vi "Load Matrix.vi"(7 "section":string, 8 "error in (no error) 2":errorcluster, 10 "refnum in":T2, 11 "Keys":string[](array[string])) -> (0 "error in (no error)":errorcluster, 1 "Matrix 2":dbl[][](array[numeric]), 2 "Matrix 1":dbl[][](array[numeric]), 3 "refnum out":T2)   [LabVIEW 2013]
uses:
  <vilib>/Utility/config.llb/Config Data RefNum.ctl
  Metadata/LBCB Number.ctl
  <vilib>/Utility/config.llb/Read Key (String).vi
  <vilib>/Utility/config.llb/NI_LVConfig.lvlib
panel:
  out "key names":string[](array[string])
  in  "LBCB Number":T1
  in  "delimiter":string="."
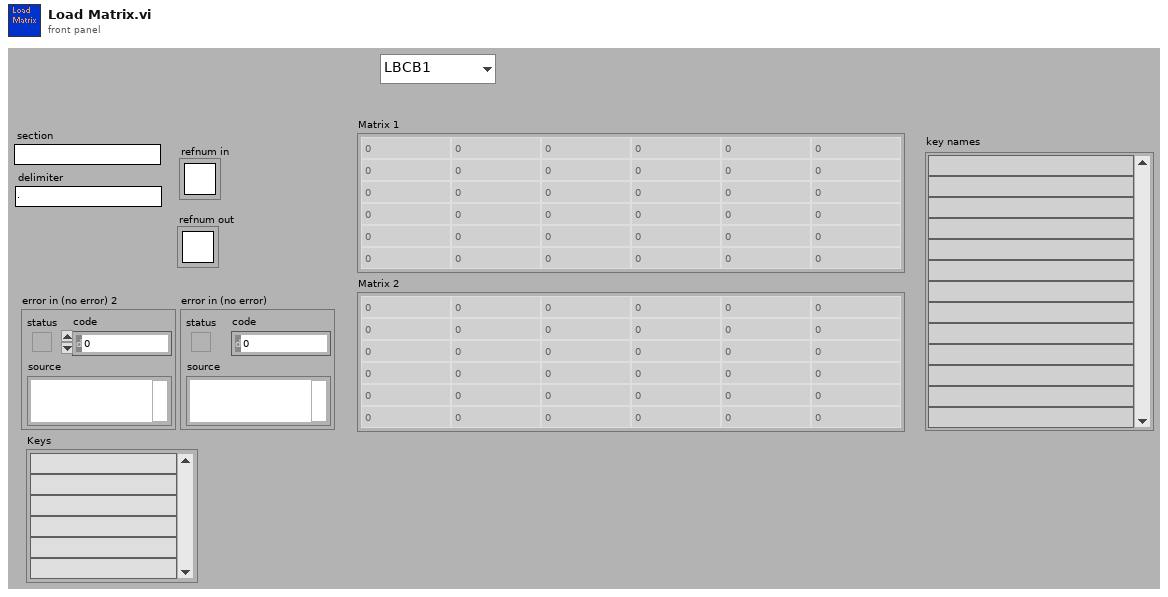
[diagram p1: front panel]
types:
  T1 = typedef "LBCB Number.ctl" = enum16{"LBCB1", "LBCB2"}
  T2 = typedef "NI_LVConfig.lvlib/Config Data RefNum.ctl" = refnum<k1>
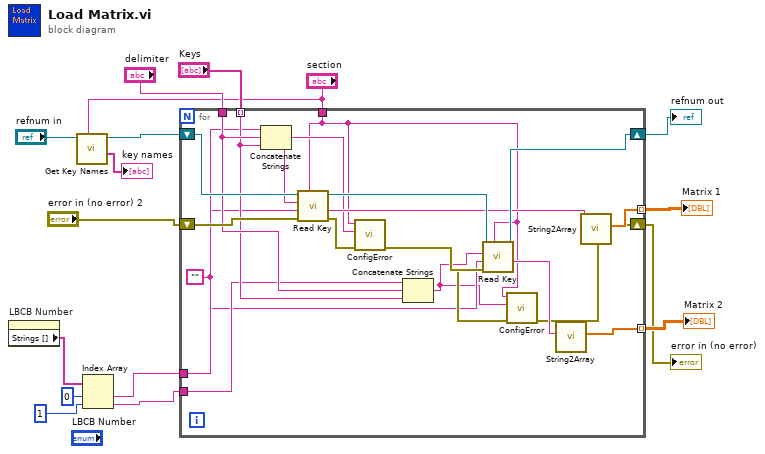
[diagram p0: block diagram]
diagram:
  n1 = property on="LBCB Number" class="Enum (strict)"() -> ("Strings []"=w8:string[])  [unwired: 2 in, 2 out]
  n2 = call <vilib>:"Get Key Names.vi"("section"="section", "refnum"="refnum in") -> ("key names"=→"key names":string[], "refnum out"=w3:T2)  [unwired: 1 in, 7 out]
  n3 = Index Array(array=w8, index #1=0 ("index"), index #2=1 ("index")) -> (element #1=w5:string, element #2=w4:string)
  n4 = for {
    tunnel: w5 -> [w19]
    tunnel: w4 -> [w20]
    shift-right: [w35] -> w10
    shift-left: w3 -> [w36]
    shift-right: [w24] -> w12
    shift-left: "error in (no error) 2" -> [w34]
    tunnel: "section" -> [w23]
    tunnel: "Keys" -> [w21] mode=indexing
    tunnel: [w31] -> w14 mode=indexing
    tunnel: [w29] -> w15 mode=indexing
    tunnel: "delimiter" -> [w22]
    w18 = ""
    n5 = Concatenate Strings(w19, w22, w21) -> (w26:string)
    n6 = call-poly <vilib>:"Read Key.vi"("section"=w23, "error in (no error)"=w34, "default value"=w18, "key"=w26, "refnum"=w36) -> ("error out"=w28:errorcluster, "value"=w30:string, "refnum out"=w33:T2)  [unwired: 1 in, 3 out]
    n7 = call "ConfigError.vi"("error in (no error)"=w28, "Key"=w26, "Section"=w23) -> ("error out"=w27:errorcluster)  [unwired: 8 out]
    n8 = Concatenate Strings(w20, w22, w21) -> (w17:string)
    n9 = call-poly <vilib>:"Read Key.vi"("section"=w23, "error in (no error)"=w27, "default value"=w18, "key"=w17, "refnum"=w33) -> ("error out"=w25:errorcluster, "value"=w32:string, "refnum out"=w35:T2)  [unwired: 1 in, 3 out]
    n10 = call "ConfigError.vi"("error in (no error)"=w25, "Key"=w17, "Section"=w23) -> ("error out"=w24:errorcluster)  [unwired: 8 out]
    n11 = call "String2Array.vi"("String"=w32) -> ("Array"=w31:dbl[])  [unwired: 1 in, 9 out]
    n12 = call "String2Array.vi"("String"=w30) -> ("Array"=w29:dbl[])  [unwired: 1 in, 9 out]
  }
  "Matrix 1" <- w15
  "Matrix 2" <- w14
  "error in (no error)" <- w12
  "refnum out" <- w10
